vi "Value Change.vi"(8 "Settings In":T1={"Step Values"=[], "Only Execute When Test Running"=TRUE, "Reset Sequence When Test Starts"=TRUE, "Current Sequence ID"=0, "Total Iterations"=0, "Current Step Start Timestamp"=0.0, "Number of Sequence Steps"=0, "Num of Analog Channels"=0, "Num of Digital Channels"=0, "Delay Before Starting Sequence"=0.0, "Show UI"=FALSE, "Time Remaining"=0.0, "Test Running"=FALSE, "Pause Timestamp"=0.0, "Default Analog Values"=[], "Default Digital Values"=[]}, 9 "Tree Data":cluster{"Tag":string[], "Settings":T3[]} {"Settings"."Data Type" items=["Tree Parent"=-1, "Numeric"=0, "String"=1, "Boolean"=2, "Enum"=3]}, 10 "Tree Tag":string, 11 "Init Refs":T5) -> (0 "Settings Out":T1={"Step Values"=[], "Only Execute When Test Running"=TRUE, "Reset Sequence When Test Starts"=TRUE, "Current Sequence ID"=0, "Total Iterations"=0, "Current Step Start Timestamp"=0.0, "Number of Sequence Steps"=0, "Num of Analog Channels"=0, "Num of Digital Channels"=0, "Delay Before Starting Sequence"=0.0, "Show UI"=FALSE, "Time Remaining"=0.0, "Test Running"=FALSE, "Pause Timestamp"=0.0, "Default Analog Values"=[], "Default Digital Values"=[]}, 3 "Tree Data out":cluster{"Tag":string[], "Settings":T3[]} {"Settings"."Data Type" items=["Tree Parent"=-1, "Numeric"=0, "String"=1, "Boolean"=2, "Enum"=3]})   [LabVIEW 2020, in "Sequencer with Output Values.lvlib" / "Sequencer with Output Values.lvclass"]
uses:
  Sequencer with Output Values.lvclass
  Control Refs.ctl
  Tree Item Settings.ctl
  Data Type.ctl
  Params.ctl
  Step Settings.ctl
  Data Type Enum.ctl
  Global Tree Data.vi
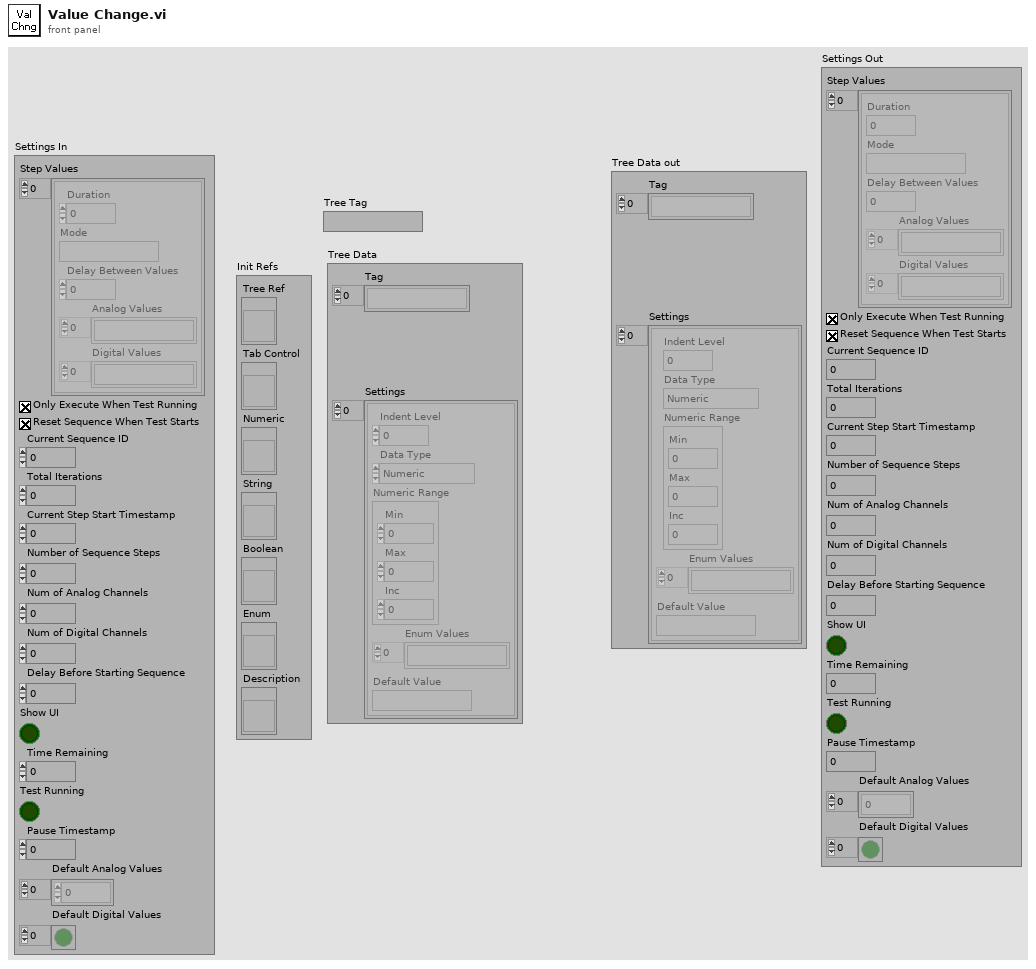
[diagram p1: front panel]
types:
  T1 = typedef "Sequencer with Output Values.lvlib/Sequencer with Output Values.lvclass/Params.ctl" = cluster{"Step Values":T2[], "Only Execute When Test Running":bool, "Reset Sequence When Test Starts":bool, "Current Sequence ID":u32, "Total Iterations":u32, "Current Step Start Timestamp":dbl, "Number of Sequence Steps":i32, "Num of Analog Channels":i32, "Num of Digital Channels":i32, "Delay Before Starting Sequence":dbl, "Show UI":bool, "Time Remaining":dbl, "Test Running":bool, "Pause Timestamp":dbl, "Default Analog Values":dbl[], "Default Digital Values":bool[]}
  T2 = typedef "Sequencer with Output Values.lvlib/Sequencer with Output Values.lvclass/Step Settings.ctl" = cluster{"Duration":dbl, "Mode":string, "Delay Between Values":dbl, "Analog Values":string[], "Digital Values":string[]}
  T3 = typedef "Sequencer with Output Values.lvlib/Sequencer with Output Values.lvclass/Tree Item Settings.ctl" = cluster{"Indent Level":i32, "Data Type":T4, "Numeric Range":cluster{"Min":dbl, "Max":dbl, "Inc":dbl}, "Enum Values":string[], "Default Value":string}
  T4 = typedef "Sequencer with Output Values.lvlib/Sequencer with Output Values.lvclass/Data Type.ctl" = i16
  T5 = typedef "Sequencer with Output Values.lvlib/Sequencer with Output Values.lvclass/Control Refs.ctl" = cluster{"Tree Ref":refnum<vi>, "Tab Control":refnum<vi>, "Numeric":refnum<vi>, "String":refnum<vi>, "Boolean":refnum<vi>, "Enum":refnum<vi>, "Description":refnum<vi>}
  T6 = typedef "Sequencer with Output Values.lvlib/Sequencer with Output Values.lvclass/Data Type Enum.ctl" = enum16{"Numeric", "String", "Boolean", "Enum"}
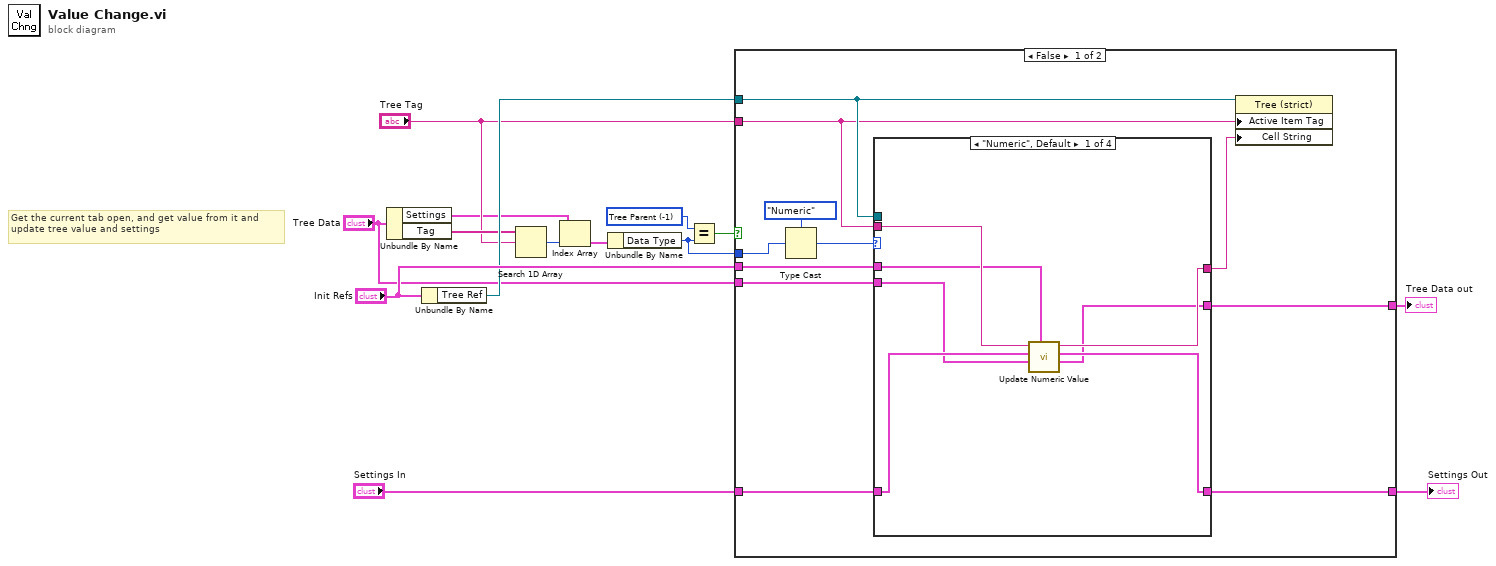
[diagram p0: block diagram]
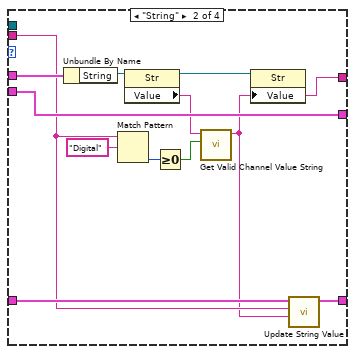
[diagram p2: hidden frame]
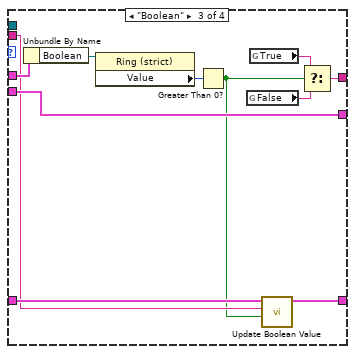
[diagram p3: hidden frame]
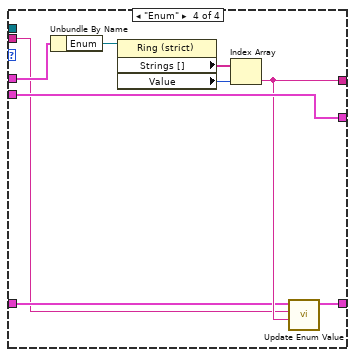
[diagram p4: hidden frame]
diagram:
  w7 = T4 -1 items=["Tree Parent"=-1, "Numeric"=0, "String"=1, "Boolean"=2, "Enum"=3, "Command"=4, "Numeric Min/Max"=5] ("Data Type")
  # "Get the current tab open, and get value from it and update tree value and settings"
  n1 = Unbundle By Name("Tree Data") -> ("Settings"=w10:T3[], "Tag"=w12:string[])
  n2 = Unbundle By Name("Init Refs") -> ("Tree Ref"=w13:refnum<vi>)
  n3 = Search 1D Array(1D array=w12, element="Tree Tag") -> (index of element=w9:i32)  [unwired: 1 in]
  n4 = Index Array(array=w10, index=w9) -> (element=w8:T3)
  n5 = Unbundle By Name(w8) -> ("Data Type"=w5:T4)
  n6 = Equal?(x=w7, y=w5) -> (x = y?=w6:bool)
  n7 = case shown="False" w6 {
    tunnel: "Init Refs" -> [w25 _]
    tunnel: w13 -> [w20 _]
    tunnel: "Tree Tag" -> [w19 _]
    tunnel: w5 -> [w24 _]
    tunnel: [w18 w66] -> w3
    tunnel: "Tree Data" -> [w17 w66]
    tunnel: "Settings In" -> [w16 w65]
    tunnel: [w15 w65] -> w1
    frame False {
      n8 = Type Cast(type=Data_Type_Enum."Numeric" ("Data Type"), x=w24) -> (*(type *) &x=w22:T6)
      n9 = case shown="\"Numeric\", Default" w22 {
        tunnel: w25 -> [w29 w44 w55 w61]
        tunnel: [w32 w33 w53 w59] -> w21
        tunnel: w20 -> [_ _ _ _]
        tunnel: w19 -> [w31 w38 w46 w56]
        tunnel: [w26 w42 w51 w64] -> w18
        tunnel: w17 -> [w27 w42 w51 w64]
        tunnel: w16 -> [w28 w41 w48 w58]
        tunnel: [w30 w40 w47 w57] -> w15
        frame "Numeric", Default {
          n10 = call "Update Numeric Value.vi"("Init Refs"=w29, "Tree Data in"=w27, "Settings In"=w28, "Tree Tag"=w31) -> ("Tree Data out"=w26:cluster{"Tag":string[], "Settings":T3[]}, "Settings In out"=w30:T1, "New Tree Value"=w32:string)  [unwired: 5 in]
        }
        frame "String" {
          n11 = Unbundle By Name(w44) -> ("String"=w43:refnum<vi>)
          n12 = Match Pattern(string=w38, regular expression="Digital") -> (offset past match=w36:i32)  [unwired: 1 in, 3 out]
          n13 = property class="Str"(reference=w43) -> (reference out=w34:refnum<vi>, "Value"=w39:string)  [unwired: 1 in, 1 out]
          n14 = Greater Or Equal To 0?(x=w36) -> (x >= 0?=w35:bool)
          n15 = call "Get Valid Channel Value String.vi"("Digital"=w35, "Channel Values"=w39) -> ("Valid Channel Values"=w33:string)  [unwired: 9 in]
          n16 = property class="Str"(reference=w34, "Value"=w33) -> ()  [unwired: 1 in, 2 out]
          n17 = call "Update String Value.vi"("Value"=w33, "Tree Tag"=w38, "Settings In"=w41) -> ("Settings Out"=w40:T1)  [unwired: 8 in]
        }
        frame "Boolean" {
          n18 = Unbundle By Name(w55) -> ("Boolean"=w54:refnum<vi>)
          n19 = property class="Ring (strict)"(reference=w54) -> ("Value"=w52:u16)  [unwired: 1 in, 2 out]
          n20 = Greater Than 0?(x=w52) -> (x > 0?=w45:bool)
          n21 = global read "Global Tree Data.vi" "False"() -> (w49:string)
          n22 = global read "Global Tree Data.vi" "True"() -> (w50:string)
          n23 = call "Update Boolean Value.vi"("Value"=w45, "Tree Tag"=w46, "Settings In"=w48) -> ("Settings Out"=w47:T1)  [unwired: 8 in]
          n24 = Select(t=w50, s=w45, f=w49) -> (s? t:f=w53:string)
        }
        frame "Enum" {
          n25 = Unbundle By Name(w61) -> ("Enum"=w60:refnum<vi>)
          n26 = property class="Ring (strict)"(reference=w60) -> ("Strings []"=w63:string[], "Value"=w62:u16)  [unwired: 1 in, 2 out]
          n27 = Index Array(array=w63, index=w62) -> (element=w59:string)
          n28 = call "Update Enum Value.vi"("Value"=w59, "Tree Tag"=w56, "Settings In"=w58) -> ("Settings Out"=w57:T1)  [unwired: 8 in]
        }
      }
      n29 = property class="Tree (strict)"(reference=w20, "Active Item Tag"=w19, "Cell String"=w21) -> ()  [unwired: 1 in, 2 out]
    }
    frame True {
    }
  }
  "Tree Data out" <- w3
  "Settings Out" <- w1
